vi "Example TIF Creation.vi"   [LabVIEW 2016]
uses:
  TIF Write Image Information.ctl
types:
  T1 = typedef "TIF Write Image Information.ctl" = cluster{"Image Width (Pixels)":u32, "Image Height (Pixels)":u32, "Pixel Width (µm)":dbl, "Pixel Height (µm)":dbl, "Bits Per Sample (e.g. 16)":u32, "No. of Frames":u32, "No. of Slices":u32, "Time Step (sec)":dbl, "Z Step (µm)":dbl}
  T2 = enum16{"big-endian, network order", "native, host order", "little-endian"}
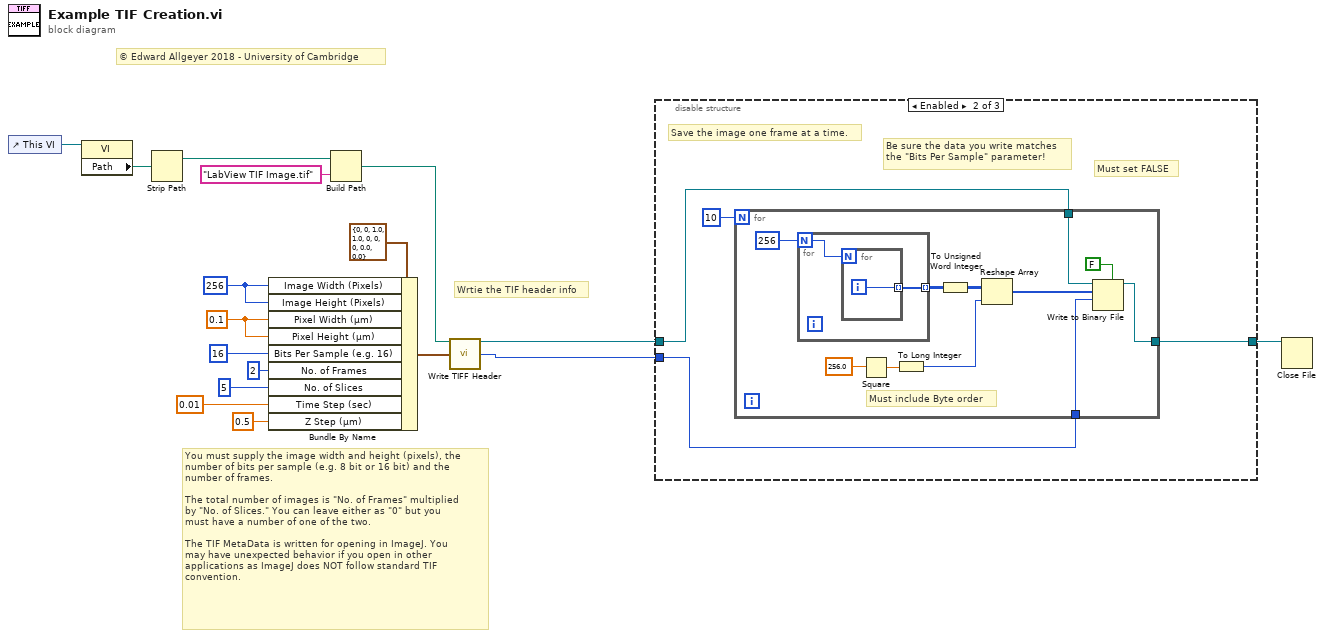
[diagram p0: block diagram]
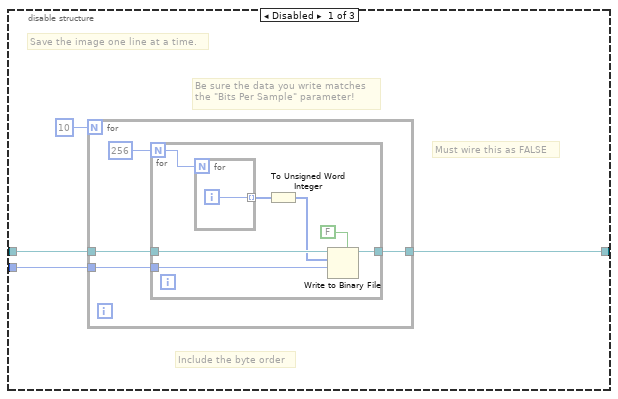
[diagram p2: hidden frame]
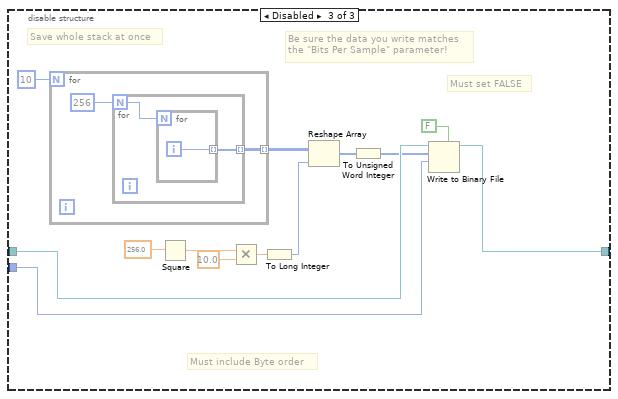
[diagram p3: hidden frame]
diagram:
  w14 = 0.1 ("Pixel Width (µm)")
  w15 = u32 256 ("Image Width (Pixels)")
  # "© Edward Allgeyer 2018 - University of Cambridge"
  # "Wrtie the TIF header info"
  # "You must supply the image width and height (pixels), the\nnumber of bits per sample (e.g. 8 bit or 16 bit) and the\nnumber of frames.\n\nThe total number of images is \"No. of Frames\" multiplied\nby \"No. of Slices.\" You can leave either as \"0\" but you\nmust have a number of one of the two.\n\nThe TIF MetaData is written for opening in ImageJ. You\nmay have unexpected behavior if you open in other\napplications as ImageJ does NOT follow standard TIF\nconvention."
  n1 = control-ref of="This VI"() -> (w8:refnum<vi>)
  n2 = property class="VI"(reference=w8) -> ("Path"=w7:path)  [unwired: 1 in, 2 out]
  n3 = Strip Path(path=w7) -> (stripped path=w6:path)  [unwired: 1 out]
  n4 = Bundle By Name(cluster=T1 {"Image Width (Pixels)"=0, "Image Height (Pixels)"=0, "Pixel Width (µm)"=1.0, "Pixel Height (µm)"=1.0, "Bits Per Sample (e.g. 16)"=0, "No. of Frames"=0, "No. of Slices"=0, "Time Step (sec)"=0.0, "Z Step (µm)"=0.0} ("Image Info"), "Image Width (Pixels)"=w15, "Image Height (Pixels)"=w15, "Pixel Width (µm)"=w14, "Pixel Height (µm)"=w14, "Bits Per Sample (e.g. 16)"=u32 16, "No. of Frames"=u32 2, "No. of Slices"=u32 5, "Time Step (sec)"=0.01, "Z Step (µm)"=0.5) -> (w16:T1)
  n5 = Build Path(base path=w6, name or relative path="LabView TIF Image.tif") -> (appended path=w4:path)
  n6 = call "Write TIFF Header.vi"("File Path"=w4, "Image Info"=w16) -> ("File Ref"=w3:refnum<file>, "Byte Order"=w2:T2)  [unwired: 11 in, 1 out]
  n7 = disable-structure shown="Enabled" {
    disable-tunnel: w3 -> [w20 w36 w54]
    disable-tunnel: w2 -> [w19 w35 w55]
    disable-tunnel: [w18 w34 w52] -> w1
    frame Disabled {
      # "Save the image one line at a time."
      # "Include the byte order"
      # "Must wire this as FALSE"
      # "Be sure the data you write matches\nthe \"Bits Per Sample\" parameter!"
      n8 = for {
        N: 10 -> [_]
        tunnel: w20 -> [w24]
        tunnel: w19 -> [w23]
        tunnel: [w22] -> w18
        n9 = for {
          N: 256 -> [w32]
          tunnel: w24 -> [w29]
          tunnel: w23 -> [w28]
          tunnel: [w27] -> w22
          n10 = for {
            N: w32 -> [_]
            tunnel: [w33] -> w31 mode=indexing
            i -> [w33]
          }
          n11 = To Unsigned Word Integer(number=w31) -> (unsigned 16bit integer=w26:u16[])
          n12 = Write to Binary File(file (use dialog)=w29, data=w26, 5:FALSE ("prepend array or string size? (T)"), 9:w28) -> (refnum out=w27:refnum<file>)  [unwired: 2 in, 2 out]
        }
      }
    }
    frame Enabled {
      # "Save the image one frame at a time."
      # "Be sure the data you write matches\nthe \"Bits Per Sample\" parameter!"
      # "Must set FALSE"
      n13 = for {
        N: 10 -> [_]
        tunnel: w36 -> [w40]
        tunnel: w35 -> [w39]
        tunnel: [w38] -> w34
        # "Must include Byte order"
        n14 = for {
          N: 256 -> [w50]
          tunnel: [w49] -> w47 mode=indexing
          n15 = for {
            N: w50 -> [_]
            tunnel: [w51] -> w49 mode=indexing
            i -> [w51]
          }
        }
        n16 = Square(x=256.0) -> (x^2=w45:dbl)
        n17 = To Long Integer(number=w45) -> (32bit integer=w43:i32)
        n18 = To Unsigned Word Integer(number=w47) -> (unsigned 16bit integer=w46:u16[][])
        n19 = Reshape Array(w46, w43) -> (w41:u16[])
        n20 = Write to Binary File(file (use dialog)=w40, data=w41, 5:FALSE ("prepend array or string size? (T)"), 9:w39) -> (refnum out=w38:refnum<file>)  [unwired: 2 in, 2 out]
      }
    }
    frame Disabled {
      # "Be sure the data you write matches\nthe \"Bits Per Sample\" parameter!"
      # "Must include Byte order"
      # "Must set FALSE"
      # "Save whole stack at once"
      n21 = for {
        N: 10 -> [_]
        tunnel: [w65] -> w61 mode=indexing
        n22 = for {
          N: 256 -> [w68]
          tunnel: [w67] -> w65 mode=indexing
          n23 = for {
            N: w68 -> [_]
            tunnel: [w69] -> w67 mode=indexing
            i -> [w69]
          }
        }
      }
      n24 = Square(x=256.0) -> (x^2=w60:dbl)
      n25 = Multiply(x=w60, y=10.0) -> (x*y=w58:dbl)
      n26 = To Long Integer(number=w58) -> (32bit integer=w57:i32)
      n27 = Reshape Array(w61, w57) -> (w56:i32[])
      n28 = To Unsigned Word Integer(number=w56) -> (unsigned 16bit integer=w53:u16[])
      n29 = Write to Binary File(file (use dialog)=w54, data=w53, 5:FALSE ("prepend array or string size? (T)"), 9:w55) -> (refnum out=w52:refnum<file>)  [unwired: 2 in, 2 out]
    }
  }
  n30 = Close File(refnum=w1) -> ()  [unwired: 1 in, 2 out]
